vi "Client Loop Async.vi"(11 "TCP Client in":refnum<class "TCP Client.lvclass">) -> ()   [LabVIEW 2012, in "Stream-TCP.lvlib" / "TCP Client.lvclass"]
uses:
  TCP Client.lvclass
  Connection State.ctl
  lv-stream/stream/Endpoint/Endpoint.lvclass
  lv-stream/stream/URI/URI.lvclass
  lv-stream/stream/Connection/Connection.lvclass
  lv-stream/stream/Connection State.ctl
  lv-stream/stream/Stream.lvlib
panel:
  out "URI String":string
  out "State":T1
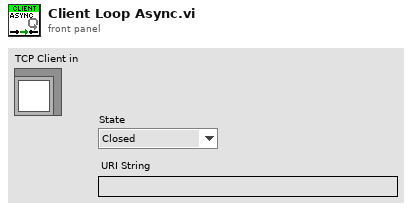
[diagram p1: front panel]
types:
  T1 = typedef "Stream-TCP.lvlib/TCP Client.lvclass/Connection State.ctl" = enum16{"Closed", "Idle", "Connecting", "Connected", "Shutdown"}
  T2 = typedef "Stream.lvlib/Connection State.ctl" = enum16{"Connected", "Disconnected"}
  T3 = typedef "Stream-TCP.lvlib/Client Command.ctl" = enum16{"Connect", "Close", "Shutdown", "Reconnect"}
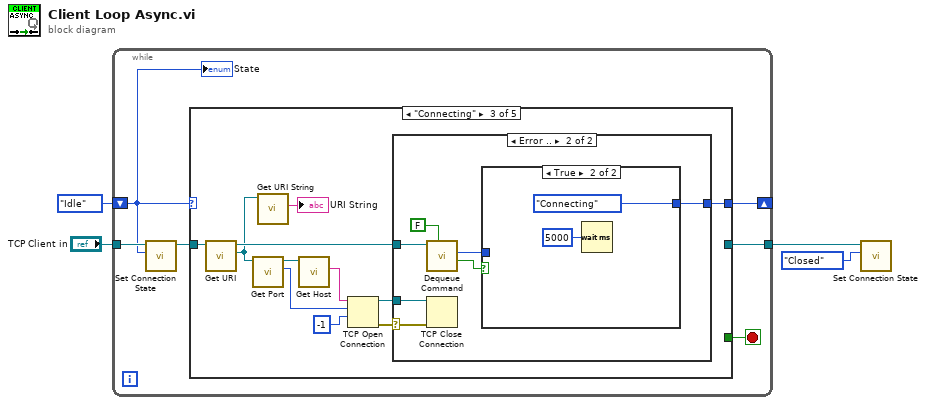
[diagram p0: block diagram]
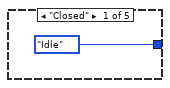
[diagram p2: hidden frame]
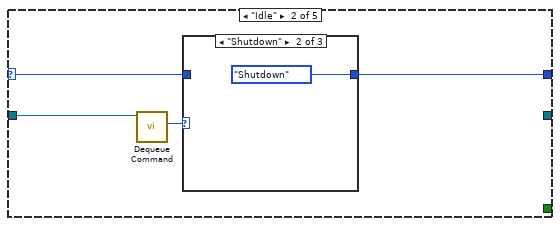
[diagram p3: hidden frame]
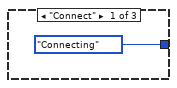
[diagram p4: hidden frame]
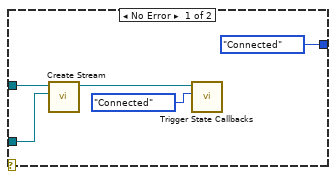
[diagram p6: hidden frame]
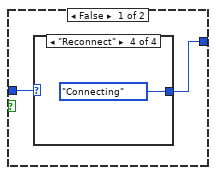
[diagram p7: hidden frame]
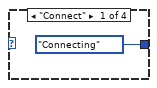
[diagram p8: hidden frame]
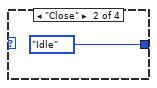
[diagram p9: hidden frame]
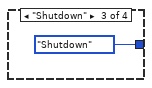
[diagram p10: hidden frame]
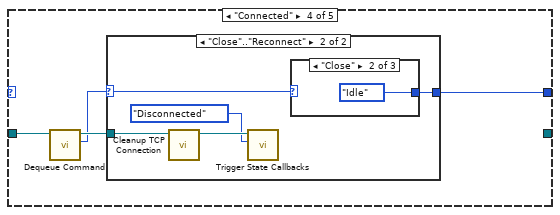
[diagram p11: hidden frame]
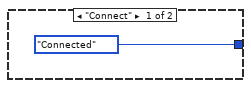
[diagram p12: hidden frame]
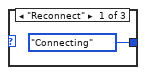
[diagram p13: hidden frame]
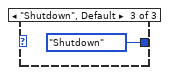
[diagram p14: hidden frame]
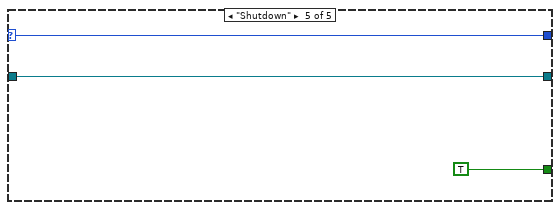
[diagram p15: hidden frame]
diagram:
  n1 = while {
    tunnel: "TCP Client in" -> [w8]
    shift-right: [w5] -> _
    shift-left: Connection_State."Idle" ("Connection State") -> [w6]
    tunnel: [w9] -> w3
    stop <- w10 stop-if-true
    n2 = call "Set Connection State.vi"("Connection State"=w6, "TCP Client in"=w8) -> ("TCP Client out"=w7:refnum<class "TCP Client.lvclass">)  [unwired: 8 in, 1 out]
    n3 = case shown="\"Connecting\"" w6 {
      selector: w6 -> [_ w13 _ _ w63]
      tunnel: [_ _ _ _ TRUE] -> w10
      tunnel: w7 -> [_ w15 w19 w52 w64]
      tunnel: [_ _ _ _ w64] -> w9
      tunnel: [Connection_State."Idle" ("Connection State") w12 w22 w53 w63] -> w5
      frame "Closed" {
      }
      frame "Idle" {
        n4 = call "Dequeue Command.vi"("TCP Client in"=w15) -> ("Command"=w14:T3)  [unwired: 7 in, 3 out]
        n5 = case shown="\"Shutdown\"" w14 {
          tunnel: [Connection_State."Connecting" ("Connection State") Connection_State."Shutdown" ("Connection State") w18] -> w12
          tunnel: w13 -> [_ _ w18]
          frame "Connect" {
          }
          frame "Shutdown" {
          }
          frame Default {
          }
        }
      }
      frame "Connecting" {
        n6 = call "Get URI.vi"("Endpoint in"=w19) -> ("URI"=w21:refnum<class "URI.lvclass">, "Endpoint out"=w24:refnum<class "TCP Client.lvclass">)  [unwired: 8 in, 1 out]
        n7 = call "Get Port.vi"("URI in"=w21) -> ("Port"=w26:u16, "URI out"=w28:refnum<class "URI.lvclass">)  [unwired: 8 in, 1 out]
        n8 = call "Get URI String.vi"("URI in"=w21) -> ("URI String"=→"URI String":string)  [unwired: 8 in, 2 out]
        n9 = call "Get Host.vi"("URI in"=w28) -> ("Host"=w27:string)  [unwired: 8 in, 2 out]
        n10 = TCP Open Connection(address=w27, remote port or service name=w26, timeout ms (60000)=-1) -> (connection ID=w23:refnum<k5>, error out=w25:errorcluster)  [unwired: 2 in]
        n11 = case shown="Error .." w25 {
          selector: w25 -> [_ w35]
          tunnel: w24 -> [w32 w40]
          tunnel: w23 -> [w31 w36]
          tunnel: [Connection_State."Connected" ("Connection State") w41] -> w22
          frame No Error {
            n12 = call "Create Stream.vi"("TCP Connection"=w31, "TCP Client in"=w32) -> ("TCP Client out"=w30:refnum<class "TCP Client.lvclass">)  [unwired: 8 in, 1 out]
            n13 = call "Trigger State Callbacks.vi"("State"=Connection_State."Connected", "Connection in"=w30) -> ()  [unwired: 8 in, 2 out]
          }
          frame Error {
            n14 = call "Dequeue Command.vi"("Wait? (T)"=FALSE, "TCP Client in"=w40) -> ("timed out?"=w38:bool, "Command"=w37:T3)  [unwired: 6 in, 2 out]
            n15 = TCP Close Connection(connection ID=w36, error in (no error)=w35) -> ()  [unwired: 1 in, 2 out]
            n16 = case shown="True" w38 {
              tunnel: [w42 Connection_State."Connecting" ("Connection State")] -> w41
              tunnel: w37 -> [w43 _]
              frame False {
                n17 = case shown="\"Reconnect\"" w43 {
                  tunnel: [Connection_State."Connecting" ("Connection State") Connection_State."Idle" ("Connection State") Connection_State."Shutdown" ("Connection State") Connection_State."Connecting" ("Connection State")] -> w42
                  frame "Connect" {
                  }
                  frame "Close" {
                  }
                  frame "Shutdown" {
                  }
                  frame "Reconnect" {
                  }
                }
              }
              frame True {
                n18 = Wait (ms)(milliseconds to wait=u32 5000) -> ()  [unwired: 1 out]
              }
            }
          }
        }
      }
      frame "Connected" {
        n19 = call "Dequeue Command.vi"("TCP Client in"=w52) -> ("Command"=w50:T3, "TCP Client out"=w51:refnum<class "TCP Client.lvclass">)  [unwired: 7 in, 2 out]
        n20 = case shown="\"Close\"..\"Reconnect\"" w50 {
          selector: w50 -> [_ w55]
          tunnel: [Connection_State."Connected" ("Connection State") w59] -> w53
          tunnel: w51 -> [_ w56]
          frame "Connect" {
          }
          frame "Close".."Reconnect" {
            n21 = call "Cleanup TCP Connection.vi"("TCP Client in"=w56) -> ("TCP Client out"=w58:refnum<class "TCP Client.lvclass">)  [unwired: 9 in, 1 out]
            n22 = call "Trigger State Callbacks.vi"("State"=Connection_State."Disconnected", "Connection in"=w58) -> ()  [unwired: 8 in, 2 out]
            n23 = case shown="\"Reconnect\"" w55 {
              tunnel: [Connection_State."Connecting" ("Connection State") Connection_State."Idle" ("Connection State") Connection_State."Shutdown" ("Connection State")] -> w59
              frame "Reconnect" {
              }
              frame "Close" {
              }
              frame "Shutdown", Default {
              }
            }
          }
        }
      }
      frame "Shutdown" {
      }
    }
    "State" <- w6
  }
  n24 = call "Set Connection State.vi"("Connection State"=Connection_State."Closed", "TCP Client in"=w3) -> ()  [unwired: 8 in, 2 out]
